vi "Read Connect Info.vi"(8 "error in (no error)":errorcluster, 11 "Motor Base in":refnum<class "Motor Base.lvclass">) -> (0 "error out":errorcluster, 2 "Connect Info":T1, 3 "Motor Base out":refnum<class "Motor Base.lvclass">)   [LabVIEW 2016, in "Motor Base.lvlib" / "Motor Base.lvclass"]
uses:
  Motor Base.lvclass
  Motor Base.lvclass/Motor Base.ctl
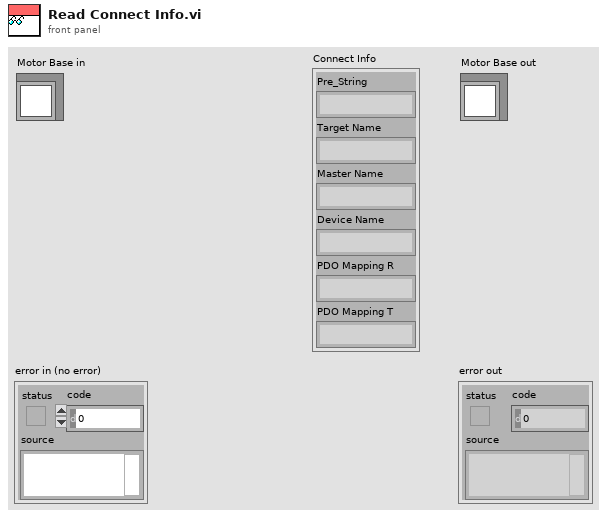
[diagram p1: front panel]
types:
  T1 = cluster{"Pre_String":string, "Target Name":string, "Master Name":string, "Device Name":string, "PDO Mapping R":string, "PDO Mapping T":string}
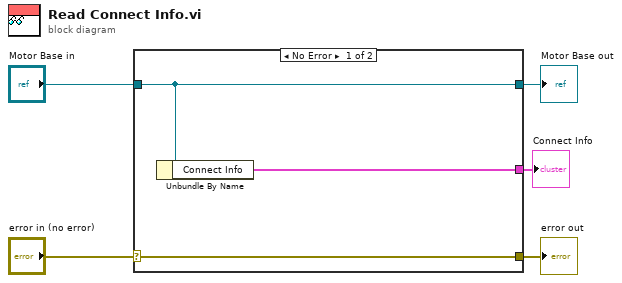
[diagram p0: block diagram]
diagram:
  n1 = case shown="No Error" "error in (no error)" {
    selector: "error in (no error)" -> [w8 w9]
    tunnel: [w8 w9] -> w4
    tunnel: [w7 w10] -> w2
    tunnel: "Motor Base in" -> [w7 w10]
    tunnel: [w6 _] -> w1
    frame No Error {
      n2 = Unbundle By Name(w7) -> ("Connect Info"=w6:T1)
    }
    frame Error {
    }
  }
  "error out" <- w4
  "Motor Base out" <- w2
  "Connect Info" <- w1
